vi "MRC Smart IO Close.vi"(8 "error in (no error)":errorcluster, 11 "deviceIndex":i32) -> (0 "error out":errorcluster)   [LabVIEW 2026, in "MrcLib.lvlib"]
doc: "MRC_Status MRC_CALLCONV MRC_SmartIO_Close(int32_t deviceIndex);"
uses:
  MrcLib.lvlib
  MrcLib.dll
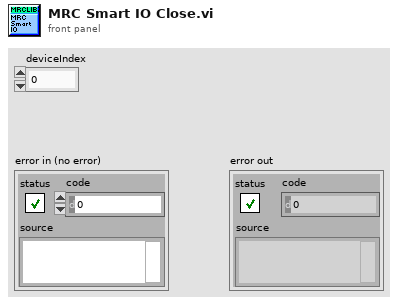
[diagram p1: front panel]
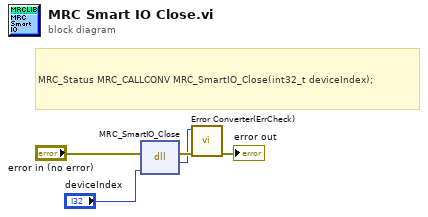
[diagram p0: block diagram]
diagram:
  # "MRC_Status MRC_CALLCONV MRC_SmartIO_Close(int32_t deviceIndex);"
  n1 = dll-call lib="MrcLib.*" fn="MRC_SmartIO_Close"(error in="error in (no error)", "deviceIndex"="deviceIndex") -> (error out=w3:errorcluster, w1:i32)  [unwired: 3 in, 1 out]
  n2 = call <vilib>:"Error Converter(ErrCheck).vi"("error in (no error)"=w3, "status"=w1) -> ("error out"=→"error out":errorcluster)  [unwired: 9 in]
